vi "subUpdateTypePaletteFile.vi"(8 "error in (no error)":errorcluster, 9 "Step Types Version":string, 11 "TypePalette .ini file location":path) -> (0 "error out":errorcluster, 3 "Type Palettes File Path out":path)   [LabVIEW 2015, in "veristand-steps-build-tools.lvlib"]
uses:
  veristand-steps-build-tools.lvlib
  <vilib>/xml/Load XML File.vi
  <vilib>/xml/Close Reference(Node).vi
  <vilib>/xml/Close Reference(NNMap).vi
  <vilib>/xml/NI_XML.lvlib
  <resource>/objmgr/DOMUserDefRef.rc
  <userlib>/Simple XML/Simple XML.lvlib
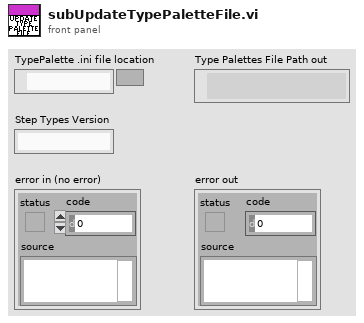
[diagram p1: front panel]
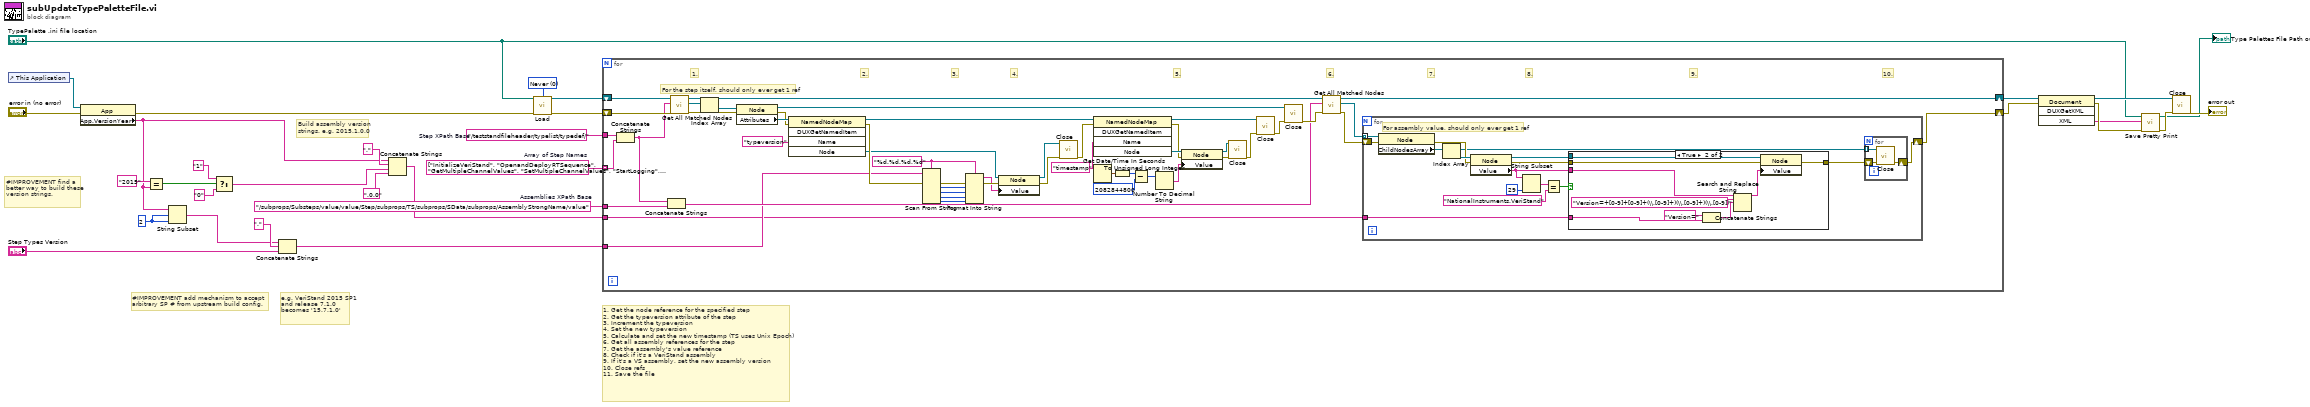
[diagram p0: block diagram]
diagram:
  w3 = 2 ("length (rest)")
  w32 = "/subprops/Substeps/value/value/Step/subprops/TS/subprops/SData/subprops/AssemblyStrongName/value"  # Assemblies XPath Base
  w30 = string[] ["InitializeVeriStand", "OpenandDeployRTSequence", "GetMultipleChannelValues", "SetMultipleChannelValues", "StartLogging", "StopLogging", "StopVeriStand", "RunProject", "ConnectProject", "DisconnectProject", "UndeployProject", "RunStimulusProfileAsynch", "DeployProject", "OpenReferences", "GetAlarmState", "SetChannelValue", "GetAlarmList", "RunStimulusProfileBlocking", "SetAlarmState", "SetModelParameterValue", "CloseProject", "UpdateModelParametersFromFile", "GetChannelValue", "LimitTestChannelValue", "GetChannelFaultValue", "GetModelParameterValue", "ClearFault", "ClearAllFaults", "PauseRTSequence", "StopRTSequence", "GetSequenceState", "GetAllSequenceNames", "StartRTSequence", "AbortRTSequence", "GetSequenceReturnValue", "StartStimulusProfileSession", "RunRTSequenceAction", "CloseWorkspace", "OpenWorkspace", "SilentConnect", "SilentDisconnect", "OpenProject", "RunRTSequencePassFail", "RunRTSequenceNumericLimit", "SetChannelFaultValue", "StopVeristandGateway", "StartVeristand", "LimitTestChannelValue_TS2014"]  # Array of Step Names
  w24 = "/teststandfileheader/typelist/typedef/"  # Step XPath Base
  w23 = 0 items=["Never", "Always", "Auto"] ("validate on load (Auto)")
  # "#IMPROVEMENT find a better way to build these version strings."
  # "Build assembly version\nstrings. e.g. 2015.1.0.0"
  # "#IMPROVEMENT add mechanism to accept\narbitrary SP # from upstream build config."
  # "e.g. VeriStand 2015 SP1 and release 7.1.0\nbecomes '15.7.1.0'"
  # "1. Get the node reference for the specified step\n2. Get the typeversion attribute of the step\n3. Increment the typeversion\n4. Set the new typeversion\n5. Calculate and set the new timestamp (TS uses Unix Epoch)\n6. Get all assembly references for the step\n7. Get the assembly's value reference\n8. Check if it's a VeriStand assembly\n9. If it's a VS assembly, set the new assembly version\n10. Close refs\n11. Save the file"
  n1 = control-ref of="This Application"() -> (w21:refnum<vi>)
  n2 = property class="App"(reference=w21, error in="error in (no error)") -> (error out=w14:errorcluster, "App.VersionYear"=w4:string)  [unwired: 1 out]
  n3 = Equal?(x="2015", y=w4) -> (x = y?=w9:bool)
  n4 = String Subset(string=w4, offset (0)=w3, length (rest)=w3) -> (substring=w2:string)
  n5 = Select(t="1" ("string"), s=w9, f="0" ("string")) -> (s? t:f=w6:string)
  n6 = Concatenate Strings(w2, "." ("string"), "Step Types Version") -> (w13:string)
  n7 = Concatenate Strings(w4, "." ("string"), w6, ".0.0" ("string")) -> (w17:string)
  n8 = call-poly <vilib>:"Load.vi"("path to XML document"="TypePalette .ini file location", "validate on load (Auto)"=w23, "error in (no error)"=w14) -> ("DOM document out"=w16:refnum<k20>, "error out"=w15:errorcluster)  [unwired: 10 in, 1 out]
  n9 = for {
    tunnel: w30 -> [w78] mode=indexing
    shift-right: [w76] -> w25
    shift-left: w16 -> [w81]
    tunnel: w24 -> [w79]
    shift-right: [w69] -> w31
    shift-left: w15 -> [w80]
    tunnel: w32 -> [w74]
    tunnel: w13 -> [w35]
    tunnel: w17 -> [w33]
    w58 = "%d.%d.%d.%d" ("format string")
    # "10."
    # "9."
    # "8."
    # "7."
    # "6."
    # "5."
    # "4."
    # "3."
    # "2."
    # "1."
    # "For the step itself, should only ever get 1 ref"
    n10 = Concatenate Strings(w79, w78) -> (w73:string)
    n11 = Concatenate Strings(w73, w74) -> (w72:string)
    n12 = call <vilib>:"Get All Matched Nodes.vi"("error in (no error)"=w80, "XPath expression"=w73, "node in"=w81) -> ("error out"=w64:errorcluster, "node result array"=w68:refnum<k20>[], "node out"=w77:refnum<k20>)  [unwired: 6 in]
    n13 = Index Array(array=w68) -> (element=w67:refnum<k20>)  [unwired: 1 in]
    n14 = property class="Node"(reference=w67, error in=w64) -> (reference out=w42:refnum<k20>, error out=w65:errorcluster, "Attributes"=w66:refnum<k20>)
    n15 = invoke class="NamedNodeMap" method="DUXGetNamedItem"(reference=w66, error in=w65, "Name"="typeversion") -> (reference out=w57:refnum<k20>, error out=w36:errorcluster, "Node"=w34:refnum<k20>)  [unwired: 2 in, 2 out]
    n16 = Scan From String(format string=w58, input string=w35, error in=w36) -> (error out=w62:errorcluster, output 1=w61:i32, output 2=w60:i32, output 3=w59:i32, output 4=w37:i32)  [unwired: 5 in, 2 out]
    n17 = Format Into String(format string=w58, error in=w62, w61, w60, w59, w37) -> (resulting string=w55:string, error out=w56:errorcluster)  [unwired: 1 in]
    n18 = property class="Node"(reference=w34, error in=w56, "Value"=w55) -> (reference out=w53:refnum<k20>, error out=w54:errorcluster)
    n19 = call-poly <vilib>:"Close.vi"("error in (no error)"=w54, "node"=w53) -> ("error out"=w52:errorcluster)  [unwired: 7 in]
    n20 = invoke class="NamedNodeMap" method="DUXGetNamedItem"(reference=w57, error in=w52, "Name"="timestamp") -> (reference out=w45:refnum<k20>, error out=w49:errorcluster, "Node"=w50:refnum<k20>)  [unwired: 2 in, 2 out]
    n21 = Get Date/Time In Seconds() -> (seconds since 1Jan1904=w41:timestamp)
    n22 = To Unsigned Long Integer(number=w41) -> (unsigned 32bit integer=w40:u32)
    n23 = Subtract(x=w40, y=u32 2082844800) -> (x-y=w38:u32)
    n24 = Number To Decimal String(number=w38) -> (decimal integer string=w48:string)  [unwired: 1 in]
    n25 = property class="Node"(reference=w50, error in=w49, "Value"=w48) -> (reference out=w46:refnum<k20>, error out=w47:errorcluster)
    n26 = call-poly <vilib>:"Close.vi"("error in (no error)"=w47, "node"=w46) -> ("error out"=w44:errorcluster)  [unwired: 7 in]
    n27 = call-poly <vilib>:"Close.vi"("error in (no error)"=w44, "named node map"=w45) -> ("error out"=w43:errorcluster)  [unwired: 7 in]
    n28 = call-poly <vilib>:"Close.vi"("error in (no error)"=w43, "node"=w42) -> ("error out"=w75:errorcluster)  [unwired: 7 in]
    n29 = call <vilib>:"Get All Matched Nodes.vi"("error in (no error)"=w75, "XPath expression"=w72, "node in"=w77) -> ("error out"=w70:errorcluster, "node result array"=w71:refnum<k20>[], "node out"=w76:refnum<k20>)  [unwired: 6 in]
    n30 = for {
      tunnel: w71 -> [w96] mode=indexing
      shift-right: [w91] -> w69
      shift-left: w70 -> [w95]
      tunnel: w33 -> [w82]
      # "For assembly value, should only ever get 1 ref"
      n31 = property class="Node"(reference=w96, error in=w95) -> (error out=w93:errorcluster, "ChildNodesArray"=w92:refnum<k20>[])  [unwired: 1 out]
      n32 = Index Array(array=w92) -> (element=w94:refnum<k20>)  [unwired: 1 in]
      n33 = property class="Node"(reference=w94, error in=w93) -> (reference out=w88:refnum<k20>, error out=w89:errorcluster, "Value"=w87:string)
      n34 = String Subset(string=w87, length (rest)=29 ("length (rest)")) -> (substring=w85:string)  [unwired: 1 in]
      n35 = Equal?(x=w85, y="NationalInstruments.VeriStand" ("Node Value 2")) -> (x = y?=w83:bool)
      n36 = case shown="True" w83 {
        tunnel: w87 -> [_ w106]
        tunnel: [w97 w102] -> w90
        tunnel: w89 -> [w97 w100]
        tunnel: w88 -> [_ w99]
        tunnel: w82 -> [_ w98]
        frame False {
        }
        frame True {
          n37 = Concatenate Strings("Version=" ("replace string (\"\")"), w98) -> (w103:string)
          n38 = Search and Replace String(input string=w106, search string="Version=+[0-9]+[0-9]+(\\.[0-9]+)(\\.[0-9]+)(\\.[0-9])", replace string=w103) -> (result string=w101:string)  [unwired: 5 in, 3 out]
          n39 = property class="Node"(reference=w99, error in=w100, "Value"=w101) -> (error out=w102:errorcluster)  [unwired: 1 out]
        }
      }
      n40 = for {
        tunnel: w92 -> [w109] mode=indexing
        shift-right: [w107] -> w91
        shift-left: w90 -> [w108]
        n41 = call-poly <vilib>:"Close.vi"("error in (no error)"=w108, "node"=w109) -> ("error out"=w107:errorcluster)  [unwired: 7 in]
      }
    }
  }
  n42 = invoke class="Document" method="DUXGetXML"(reference=w25, error in=w31) -> (reference out=w28:refnum<k20>, error out=w27:errorcluster, "XML"=w26:string)  [unwired: 2 in, 1 out]
  n43 = call <userlib>:"Save Pretty Print.vi"("error in (no error)"=w27, "Pretty XML String"=w26, "XML file path"="TypePalette .ini file location") -> ("error out"=w29:errorcluster, "XML file path out"=→"Type Palettes File Path out":path)  [unwired: 7 in]
  n44 = call-poly <vilib>:"Close.vi"("error in (no error)"=w29, "node"=w28) -> ("error out"=→"error out":errorcluster)  [unwired: 7 in]
